vi "Get XY Scale Properties from Variant.vi"(8 "error in (no error)":errorcluster, 10 "Use Defaults":bool, 11 "variant":variant) -> (0 "error out":errorcluster, 2 "Scale Properties":T1 {"X.Format" items=["Decimal", "Scientific", "Engineering", "Binary", "Octal", "Hexadecimal", "Relative Time", "Time and Date", "SI", "Automatic"]; "Y.Precision:" items=["0", "1", "2", "3", "4", "5", "6", "7"]; "Y.Format" items=["Decimal", "Scientific", "Engineering", "Binary", "Octal", "Hexadecimal", "Relative Time", "Time and Date", "SI", "Automatic"]; "X.Precision" items=["0", "1", "2", "3", "4", "5", "6", "7"]}, 3 "variant dup":variant)   [LabVIEW 2012, in "Workspace MultiY Graph.lvlib"]
uses:
  Workspace MultiY Graph.lvlib
  XY Scale Properties.ctl
  XY Scale Precision.ctl
  XY Scale Format.ctl
panel:
  in  "ScalePropsFromVar":T1 {"X.Format" items=["Decimal", "Scientific", "Engineering", "Binary", "Octal", "Hexadecimal", "Relative Time", "Time and Date", "SI", "Automatic"]; "Y.Precision:" items=["0", "1", "2", "3", "4", "5", "6", "7"]; "Y.Format" items=["Decimal", "Scientific", "Engineering", "Binary", "Octal", "Hexadecimal", "Relative Time", "Time and Date", "SI", "Automatic"]; "X.Precision" items=["0", "1", "2", "3", "4", "5", "6", "7"]}
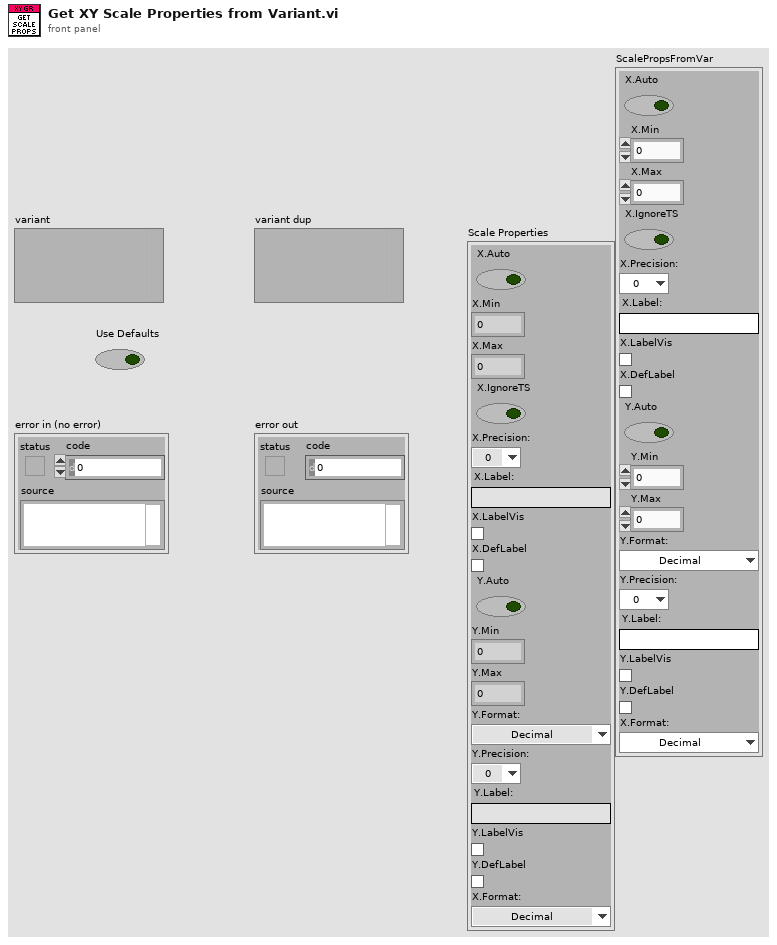
[diagram p1: front panel]
types:
  T1 = typedef "Workspace MultiY Graph.lvlib/XY Scale Properties.ctl" = cluster{"X.Auto":bool, "X.Min":dbl, "X.Max":dbl, "X.IgnoreTS":bool, "X.Precision":T2, "X.Label:":string, "X.LabelVis":bool, "X.DefLabel":bool, "Y.Auto":bool, "Y.Min":dbl, "Y.Max":dbl, "Y.Format":T3, "Y.Precision:":T2, "Y.Label:":string, "Y.LabelVis":bool, "Y.DefLabel":bool, "X.Format":T3}
  T2 = typedef "Workspace MultiY Graph.lvlib/XY Scale Precision.ctl" = u8
  T3 = typedef "Workspace MultiY Graph.lvlib/XY Scale Format.ctl" = u8
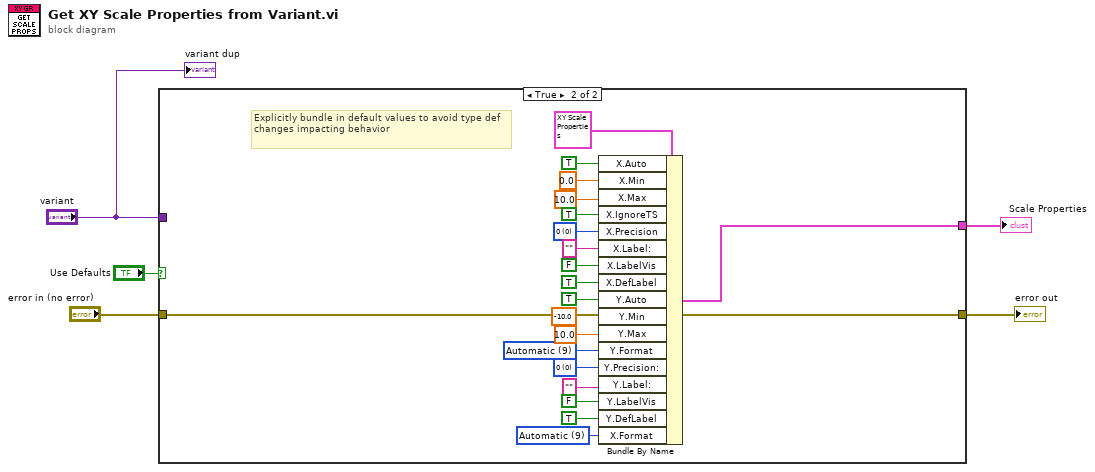
[diagram p0: block diagram]
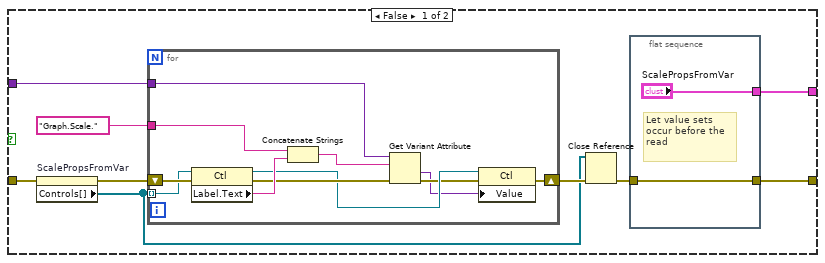
[diagram p2: hidden frame]
diagram:
  n1 = case shown="True" "Use Defaults" {
    tunnel: "error in (no error)" -> [w14 w45]
    tunnel: [w7 w45] -> w4
    tunnel: "variant" -> [w10 _]
    tunnel: [w8 w46] -> w1
    frame False {
      n2 = property on="ScalePropsFromVar" class="Clust (strict)"(error in=w14) -> (error out=w13:errorcluster, "Controls[]"=w11:refnum<vi>[])  [unwired: 1 in, 1 out]
      n3 = for {
        tunnel: w11 -> [w26] mode=indexing
        tunnel: "Graph.Scale." ("name") -> [w24]
        shift-right: [w25] -> w12
        shift-left: w13 -> [w27]
        tunnel: w10 -> [w23]
        n4 = property on="Property Node" class="Ctl"(reference=w26, error in=w27) -> (reference out=w19:refnum<vi>, error out=w21:errorcluster, "Label.Text"=w22:string)
        n5 = Concatenate Strings(w24, w22) -> (w20:string)
        n6 = Get Variant Attribute(Variant=w23, name=w20, error in=w21) -> (value=w17:variant, error out=w18:errorcluster)  [unwired: 1 in, 2 out]
        n7 = property on="Property Node" class="Ctl"(reference=w19, error in=w18, "Value"=w17) -> (error out=w25:errorcluster)  [unwired: 1 out]
      }
      n8 = Close Reference(reference=w11, error in (no error)=w12) -> (error out=w6:errorcluster)
      n9 = flat-sequence {
        tunnel: ["ScalePropsFromVar"] -> w8
        tunnel: [w15] -> w7
        tunnel: w6 -> [w15]
        frame #0 {
          # "Let value sets occur before the read"
        }
      }
    }
    frame True {
      w28 = T3 9 items=["Decimal", "Scientific", "Engineering", "Binary", "Octal", "Hexadecimal", "Relative Time", "Time and Date", "SI", "Automatic"] ("X.Format")
      w32 = T2 0 items=["0", "1", "2", "3", "4", "5", "6", "7"] ("X.Precision 2")
      w33 = T3 9 items=["Decimal", "Scientific", "Engineering", "Binary", "Octal", "Hexadecimal", "Relative Time", "Time and Date", "SI", "Automatic"] ("Y.Format")
      w40 = T2 0 items=["0", "1", "2", "3", "4", "5", "6", "7"] ("X.Precision")
      # "Explicitly bundle in default values to avoid type def changes impacting behavior"
      n10 = Bundle By Name(cluster=T1 {"X.Auto"=FALSE, "X.Min"=0.0, "X.Max"=0.0, "X.IgnoreTS"=FALSE, "X.Precision"=0, "X.Label:"="", "X.LabelVis"=FALSE, "X.DefLabel"=FALSE, "Y.Auto"=FALSE, "Y.Min"=0.0, "Y.Max"=0.0, "Y.Format"=0, "Y.Precision:"=0, "Y.Label:"="", "Y.LabelVis"=FALSE, "Y.DefLabel"=FALSE, "X.Format"=0} ("Scale Properties"), "X.Auto"=TRUE, "X.Min"=0.0, "X.Max"=10.0, "X.IgnoreTS"=TRUE, "X.Precision"=w40, "X.Label:"="" ("X.Label"), "X.LabelVis"=FALSE ("X.Label.Visible"), "X.DefLabel"=TRUE ("X.Label.Default"), "Y.Auto"=TRUE, "Y.Min"=-10.0, "Y.Max"=10.0, "Y.Format"=w33, "Y.Precision:"=w32, "Y.Label:"="" ("X.Label 2"), "Y.LabelVis"=FALSE ("X.Label.Visible 2"), "Y.DefLabel"=TRUE ("X.Label.Default 2"), "X.Format"=w28) -> (w46:T1)
    }
  }
  "error out" <- w4
  "Scale Properties" <- w1
  "variant dup" <- "variant"
